vi "Copy.vi"(0 "Subroutine in":refnum<class "Subroutine.lvclass">, 1 "Linked List Ref":refnum<data-value>, 2 "New Parent ID":string, 5 "Test ID":string, 7 "Insertion Index":i32=-1, 9 "Move?":bool, 11 "error in (no error)":errorcluster, 12 "New ID":string, 13 "Data IDs":variant) -> (3 "Linked List Ref out":refnum<data-value>, 6 "Linked List ID out":string, 14 "Data IDs out":variant, 15 "error out":errorcluster)   [LabVIEW 2020, in "Test Executive.lvlib" / "Subroutine.lvclass"]
uses:
  <vilib>/gpm_packages/@cs/test-executive/Source/Test Executive/Subroutine/Subroutine.lvclass
  <vilib>/gpm_packages/@cs/linked-list/Source/Linked List/ILinkedList/ILinked List.lvclass
  <vilib>/gpm_packages/@cs/linked-list/Source/Linked List/Linked List Ref/Linked List Ref.lvclass
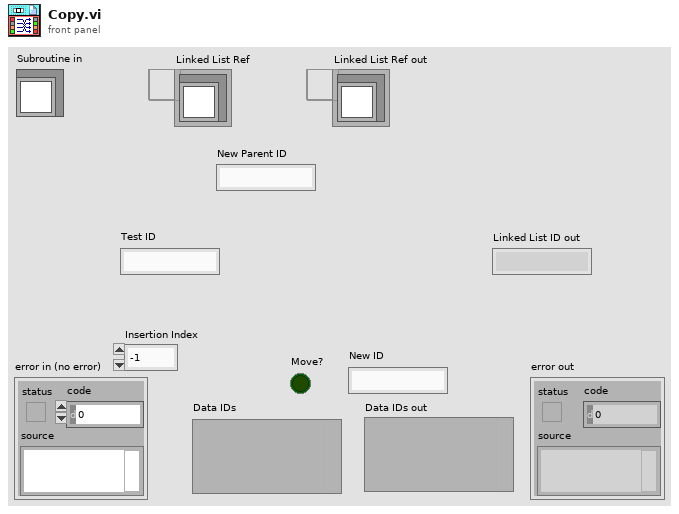
[diagram p1: front panel]
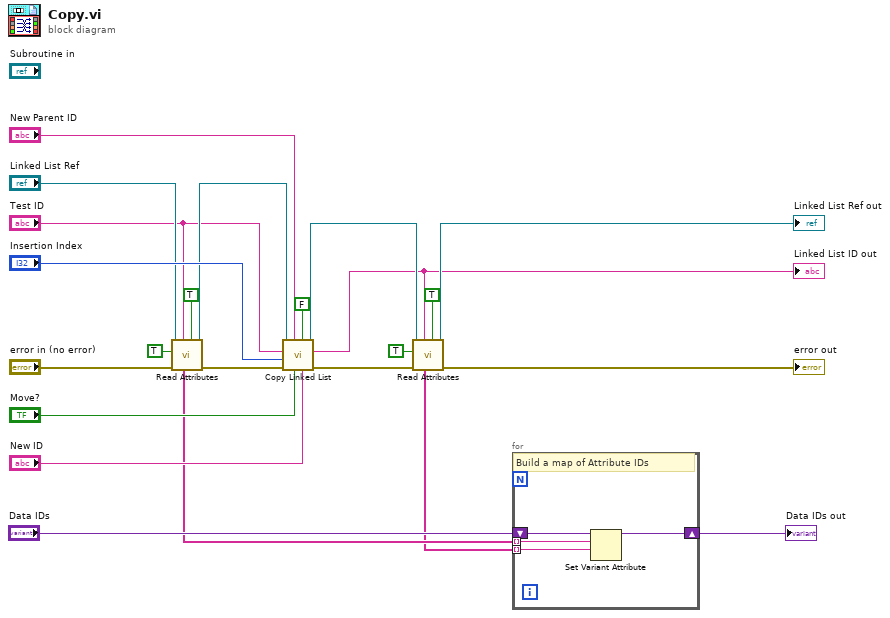
[diagram p0: block diagram]
diagram:
  n1 = call <vilib>:"Read Attributes.vi"("Flatten Pointer?"=TRUE, "Linked List ID"="Test ID", "error in (no error)"="error in (no error)", "Include Private?"=TRUE, "Linked List Ref"="Linked List Ref") -> ("error out"=w8:errorcluster, "Linked List Ref out"=w6:refnum<data-value>, "Data IDs"=w2:string[])  [unwired: 1 in, 3 out]
  n2 = call <vilib>:"Copy Linked List.vi"("New Linked List ID"="New ID", "Recursive? (T)"=FALSE, "Move?"="Move?", "New Parent Linked List ID"="New Parent ID", "error in (no error)"=w8, "Insertion Index"="Insertion Index", "Linked List ID"="Test ID", "Linked List Ref"=w6) -> ("error out"=w16:errorcluster, "Linked List ID out"=w12:string, "Linked List Ref out"=w14:refnum<data-value>)  [unwired: 1 out]
  "Linked List ID out" <- w12
  n3 = call <vilib>:"Read Attributes.vi"("Flatten Pointer?"=TRUE, "Linked List ID"=w12, "error in (no error)"=w16, "Include Private?"=TRUE, "Linked List Ref"=w14) -> ("error out"=→"error out":errorcluster, "Linked List Ref out"=→"Linked List Ref out":refnum<data-value>, "Data IDs"=w1:string[])  [unwired: 1 in, 3 out]
  n4 = for {
    tunnel: w2 -> [w26] mode=indexing
    tunnel: w1 -> [w25] mode=indexing
    shift-right: [w24] -> w3
    shift-left: "Data IDs" -> [w27]
    # "Build a map of Attribute IDs"
    n5 = Set Variant Attribute(Variant=w27, name=w26, value=w25) -> (Variant out=w24:variant)  [unwired: 1 in, 2 out]
  }
  "Data IDs out" <- w3
